vi "Write Add Scrubber.vi"(8 "error in":errorcluster, 10 "Add Scrubber":refnum<class "Scrubber.lvclass">, 11 "Options in":refnum<class "Options.lvclass">) -> (0 "error out":errorcluster, 3 "Options out":refnum<class "Options.lvclass">)   [LabVIEW 2020, in "Approval Tests.lvlib" / "Options.lvclass"]
uses:
  Options.lvclass
  Scrubber/Scrubber.lvclass
  Options.lvclass/Options.ctl
  Multi Scrubber/Multi Scrubber.lvclass
  C:/Users/SAS/Desktop/ApprovalTests.LabVIEW/Source/Approval Tests/Scrubber/Scrubber.lvclass
  Multi Scrubber/Multi Scrubber.lvclass/Multi Scrubber.ctl
  Multi Scrubber/Read Scrubbers.vi
  Multi Scrubber/Write Scrubbers.vi
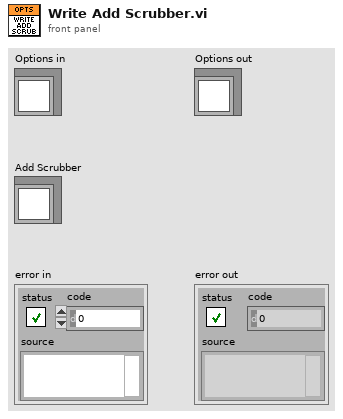
[diagram p1: front panel]
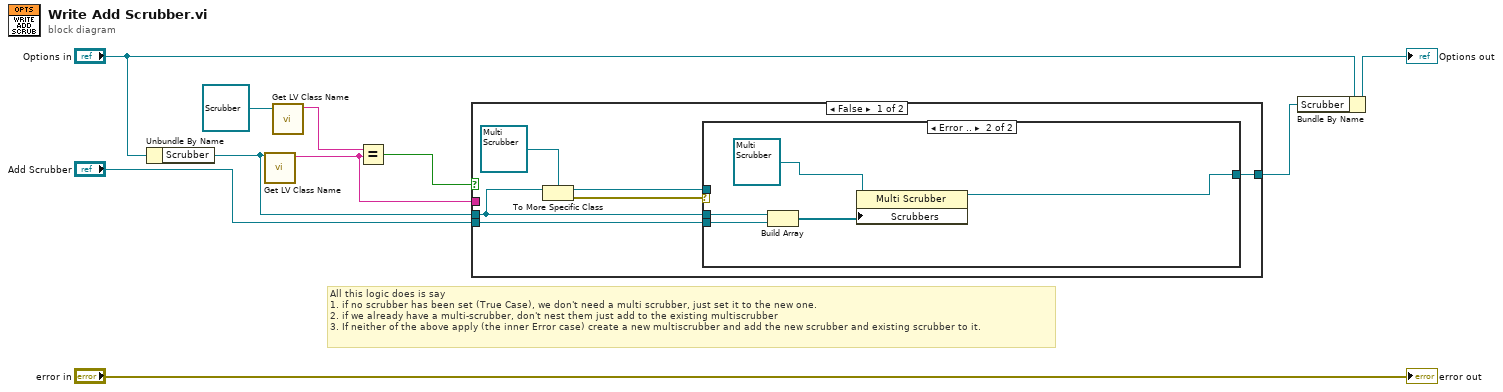
[diagram p0: block diagram]
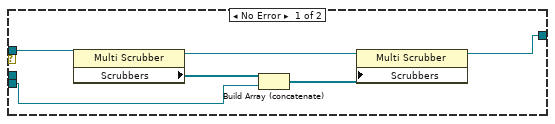
[diagram p2: hidden frame]
diagram:
  # "All this logic does is say \n1. if no scrubber has been set (True Case), we don't need a multi scrubber, just set it to the new one.\n2. if we already have a multi-scrubber, don't nest them just add to the existing multiscrubber\n3. If neither of the above apply (the inner Error case) create a new multiscrubber and add the new scrubber and existing scrubber to it."
  n1 = Unbundle By Name("Options in") -> ("Scrubber"=w4:refnum<class "Scrubber.lvclass">)
  n2 = call <vilib>:"Get LV Class Name.vi"("object"=w4) -> ("class name"=w1:string)  [unwired: 9 in, 1 out]
  n3 = call <vilib>:"Get LV Class Name.vi"("object"=refnum<class "Scrubber.lvclass"> refnum ("Approval Tests.lvlib:Scrubber.lvclass")) -> ("class name"=w3:string)  [unwired: 9 in, 1 out]
  n4 = Equal?(x=w3, y=w1) -> (x = y?=w2:bool)
  n5 = case shown="False" w2 {
    tunnel: [w15 w28] -> w8
    tunnel: "Add Scrubber" -> [w14 w28]
    tunnel: w4 -> [w12 _]
    tunnel: w1 -> [_ _]
    frame False {
      n6 = To More Specific Class(target class=refnum<class "Multi Scrubber.lvclass"> refnum ("Approval Tests.lvlib:Multi Scrubber.lvclass"), reference=w12) -> (specific class reference=w11:refnum<class "Multi Scrubber.lvclass">, error out=w16:errorcluster)  [unwired: 1 in]
      n7 = case shown="Error .." w16 {
        tunnel: [w17 w26] -> w15
        tunnel: w14 -> [w20 w24]
        tunnel: w12 -> [_ w23]
        tunnel: w11 -> [w22 _]
        frame No Error {
          n8 = property class="Multi Scrubber"(reference=w22) -> (reference out=w18:refnum<class "Multi Scrubber.lvclass">, "Scrubbers"=w21:refnum<class "Scrubber.lvclass">[])  [unwired: 1 in, 1 out]
          n9 = Build Array (concatenate)(w21, w20) -> (w19:refnum<class "Scrubber.lvclass">[])
          n10 = property class="Multi Scrubber"(reference=w18, "Scrubbers"=w19) -> (reference out=w17:refnum<class "Multi Scrubber.lvclass">)  [unwired: 1 in, 1 out]
        }
        frame Error {
          n11 = Build Array(w23, w24) -> (w25:refnum<class "Scrubber.lvclass">[])
          n12 = property class="Multi Scrubber"(reference=refnum<class "Multi Scrubber.lvclass"> refnum ("Approval Tests.lvlib:Multi Scrubber.lvclass"), "Scrubbers"=w25) -> (reference out=w26:refnum<class "Multi Scrubber.lvclass">)  [unwired: 1 in, 1 out]
        }
      }
    }
    frame True {
    }
  }
  n13 = Bundle By Name(cluster="Options in", "Scrubber"=w8) -> (→"Options out":refnum<class "Options.lvclass">)
  "error out" <- "error in"
